vi "TupnOn.vi"(11 "Pump_1AI_1DO_2DI in":refnum<class "PM_Group.lvclass">) -> (3 "Pump_1AI_1DO_2DI out":refnum<class "PM_Group.lvclass">)   [LabVIEW 2019, in "PM_Group.lvclass"]
uses:
  PM_Group.lvclass
  TypeDef/StatePump.ctl
  FPGA_API_class/FPGA API.lvclass
panel:
  out "error out":errorcluster
  in  "error in (no error)":errorcluster
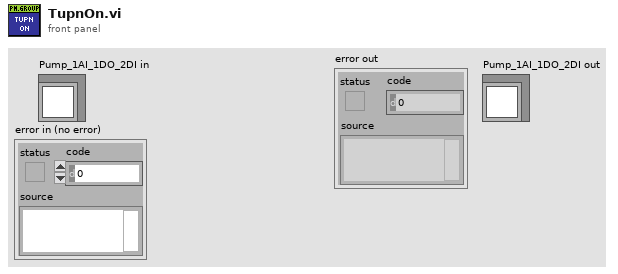
[diagram p1: front panel]
types:
  T1 = typedef "StatePump.ctl" = enum16{"Off", "TupningOn", "On", "TurningOff"}
  T2 = typedef "DO index.ctl" = u8
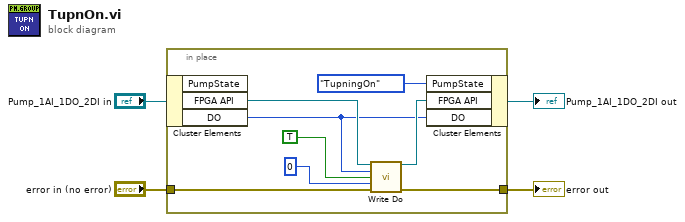
[diagram p0: block diagram]
diagram:
  n1 = in-place {
    in-place-border: [w6] -> w2
    in-place-border: "error in (no error)" -> [w5]
    n2 = in-place-cluster #1("Pump_1AI_1DO_2DI in") -> ("FPGA API"=w10:refnum<class "FPGA API.lvclass">, "DO"=w8:T2)  [unwired: 1 out]
    n3 = call "Write Do.vi"("FPGA API in"=w10, "#DO"=w8, "value"=TRUE, "Time uSec"=u32 0, "error in (no error)"=w5) -> ("FPGA API out"=w9:refnum<class "FPGA API.lvclass">, "error out"=w6:errorcluster)  [unwired: 9 in]
    n4 = in-place-cluster #1("PumpState"=StatePump."TupningOn", "FPGA API"=w9, "DO"=w8) -> (→"Pump_1AI_1DO_2DI out":refnum<class "PM_Group.lvclass">)
  }
  "error out" <- w2
